vi "WrapValue.vi"(6 "wrap_range":fxp<+/-,32,4>, 8 "Input valid":bool, 9 "wrap_min":fxp<+/-,32,4>, 10 "wrap_max":fxp<+/-,32,4>, 11 "x_in":fxp<+/-,32,4>) -> (0 "output valid":bool, 3 "x_out":fxp<+/-,32,4>)   [LabVIEW 2013]
uses:
  <vilib>/rvi/FXPMathLib/FxpSub/XNode/nifxpmath_Sub.xnode
  <vilib>/rvi/FXPMathLib/FxpAdd/XNode/nifxpmath_Add.xnode
  <vilib>/rvi/FXPMathLib/sim/FxpSim.dll
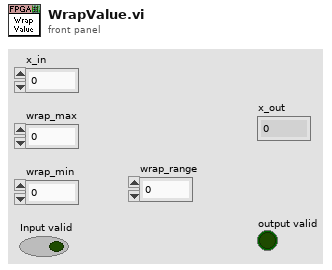
[diagram p1: front panel]
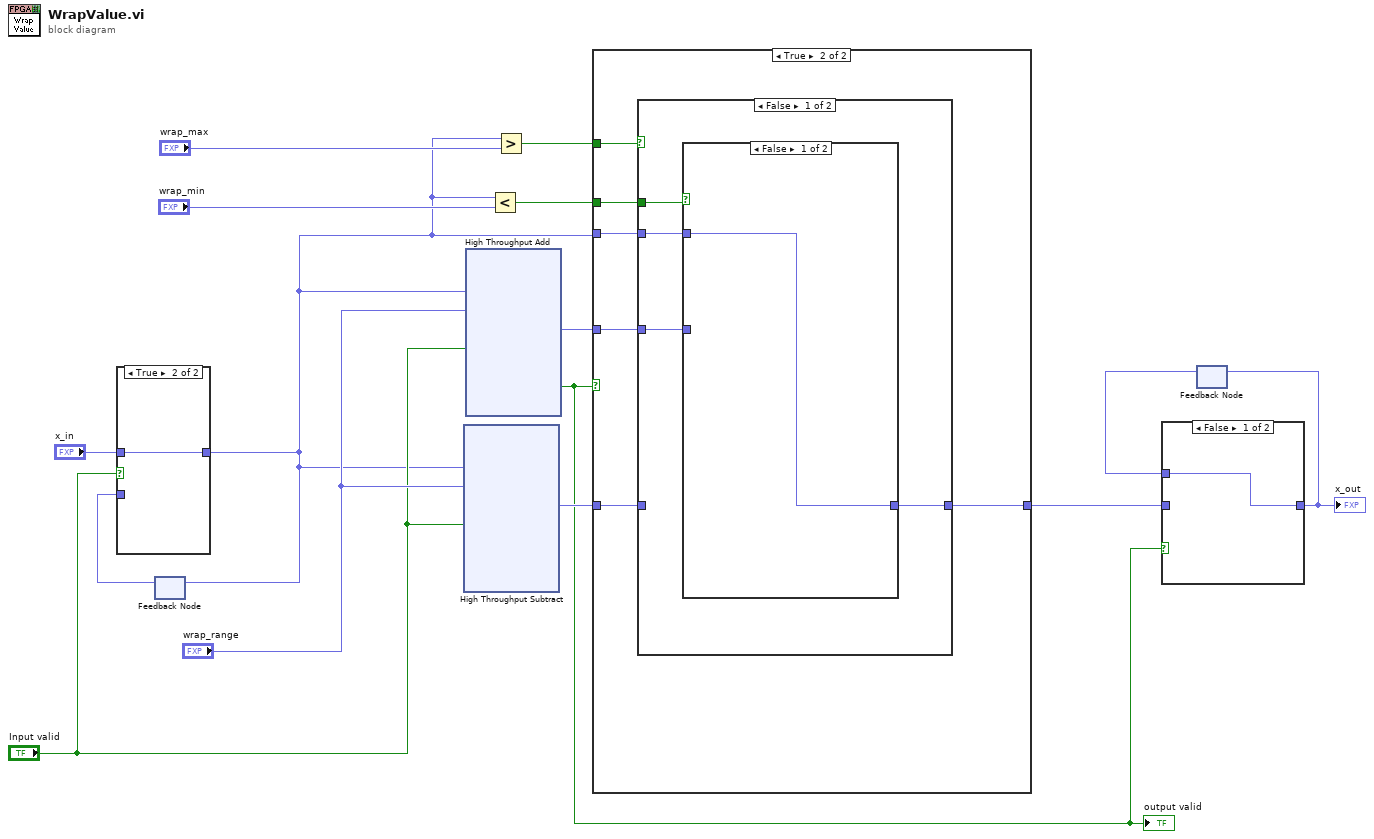
[diagram p0: block diagram]
diagram:
  n1 = feedback #1() -> (w6:fxp<+/-,32,4>)  [unwired: 1 in]
  n2 = case shown="True" "Input valid" {
    tunnel: [w16 w17] -> w1
    tunnel: "x_in" -> [_ w17]
    tunnel: w6 -> [w16 _]
    frame False {
    }
    frame True {
    }
  }
  n3 = feedback-in #1(w1) -> ()
  n4 = xnode "High Throughput Subtract"("x"=w1, "y"="wrap_range", "input valid"="Input valid") -> ("x-y"=w10:fxp<+/-,32,4>)  [unwired: 1 in, 2 out]
  n5 = xnode "High Throughput Add"("x"=w1, "y"="wrap_range", "input valid"="Input valid") -> ("x+y"=w11:fxp<+/-,32,4>, "output valid"=w5:bool)  [unwired: 1 in, 1 out]
  "output valid" <- w5
  n6 = Less?(x=w1, y="wrap_min") -> (x < y?=w9:bool)
  n7 = Greater?(x=w1, y="wrap_max") -> (0:w12:bool)
  n8 = case shown="True" w5 {
    tunnel: w12 -> [_ w24]
    tunnel: w11 -> [_ w23]
    tunnel: w10 -> [_ w22]
    tunnel: [w18 w21] -> w4
    tunnel: w9 -> [_ w20]
    tunnel: w1 -> [w18 w19]
    frame False {
    }
    frame True {
      n9 = case shown="False" w24 {
        tunnel: w23 -> [w26 _]
        tunnel: w22 -> [_ w31]
        tunnel: [w27 w31] -> w21
        tunnel: w20 -> [w28 _]
        tunnel: w19 -> [w25 _]
        frame False {
          n10 = case shown="False" w28 {
            tunnel: [w29 w30] -> w27
            tunnel: w26 -> [_ w30]
            tunnel: w25 -> [w29 _]
            frame False {
            }
            frame True {
            }
          }
        }
        frame True {
        }
      }
    }
  }
  n11 = feedback #2() -> (w2:fxp<+/-,32,4>)  [unwired: 1 in]
  n12 = case shown="False" w5 {
    tunnel: [w32 w33] -> w3
    tunnel: w4 -> [_ w33]
    tunnel: w2 -> [w32 _]
    frame False {
    }
    frame True {
    }
  }
  "x_out" <- w3
  n13 = feedback-in #2(w3) -> ()
